vi "controllerMain.vi"(8 "error in (no error)":errorcluster, 10 "UserEvents in":refnum<class "UserEvents.lvclass">, 11 "Controller in":refnum<class "Controller.lvclass">) -> (0 "error out":errorcluster, 3 "Controller out":refnum<class "Controller.lvclass">)   [LabVIEW 2015, in "Controller.lvclass"]
uses:
  Controller.lvclass
  UserEvents/UserEvents.lvclass
  StateFactory/StateFactory.lvclass
  Typedefs/StateSelector.ctl
  Model/Model/Model.lvclass
  Context/Context.lvclass
  CommandFactory/CommandFactory.lvclass
  <userlib>/Common/SerialProtocols/SerialProtocolFactory/SerialProtocolFactory/SerialProtocolFactory.lvclass
  <userlib>/Common/SerialProtocols/SerialCommunicator/SerialCommunicator.lvclass
  Model/ILCTC/ILCTC.lvclass
  Model/PressureSensor/PressureSensor/PressureSensor.lvclass
  <userlib>/Common/SerialProtocols/SerialCommunicator/SerialCommunicator.lvclass/SerialCommunicator.ctl
  <userlib>/Common/ILC/ILC/ILC.lvclass/ILC.ctl
  Model/Model/Model.lvclass/Model.ctl
  UserEvents/UserEvents.lvclass/UserEvents.ctl
  Context/Context.lvclass/Context.ctl
  Command/Command.lvclass
  Typedefs/FAMTTypedefs.lvlib
  <userlib>/Common/ILC/ILC/ILC.lvclass
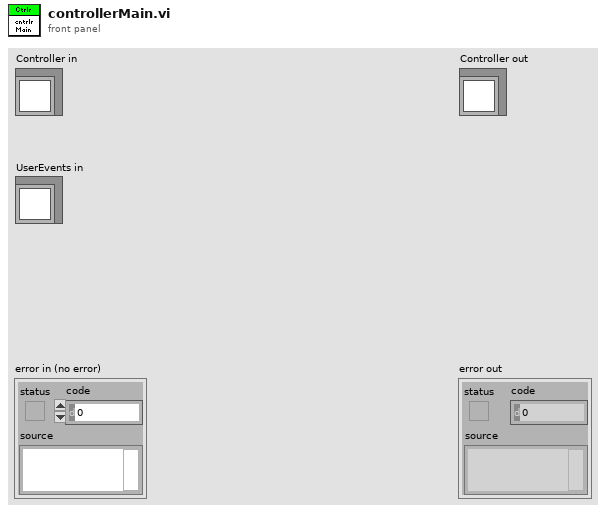
[diagram p1: front panel]
types:
  T1 = typedef "FAMTTypedefs.lvlib/StateSelector.ctl" = enum16{"OfflineState", "FaultState", "StandbyState", "DisabledState", "EnabledState", "WaitForUserInputState", "PerformOpenLoopScanState"}
  T2 = typedef "FAMTTypedefs.lvlib/SubDataEvents.ctl" = cluster{"Command":refnum<user-event>}
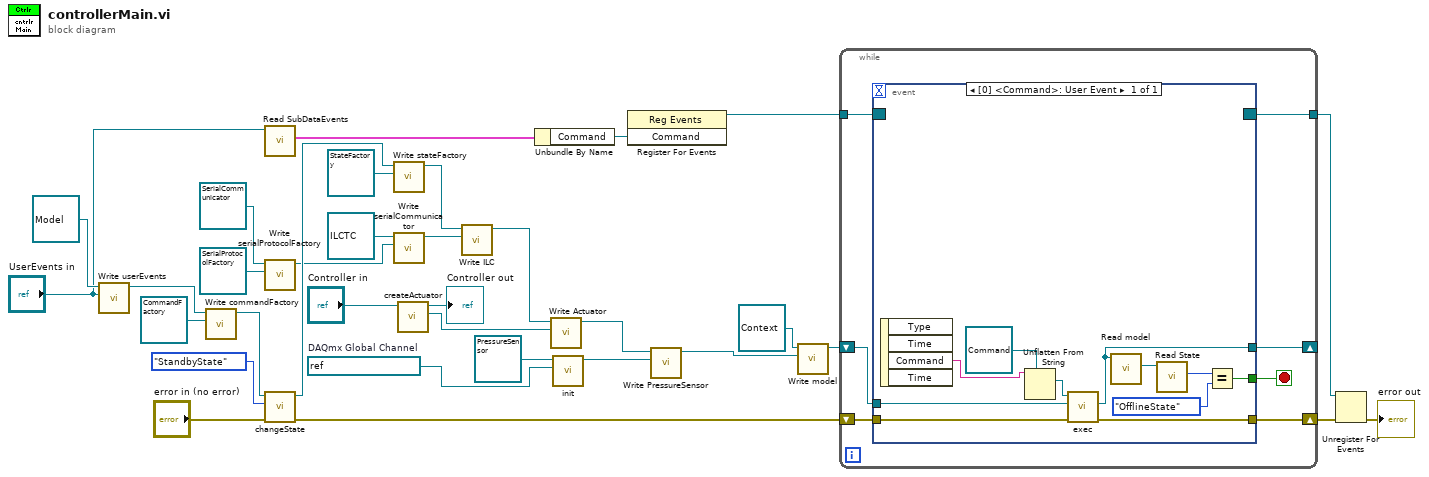
[diagram p0: block diagram]
diagram:
  w1 = refnum<k21> "PressureSensor1"  # DAQmx Global Channel
  n1 = call "Write userEvents.vi"("userEvents"="UserEvents in", "Model in"=refnum<class "Model.lvclass"> refnum) -> ("Model out"=w17:refnum<class "Model.lvclass">)  [unwired: 9 in]
  n2 = call "Write commandFactory.vi"("commandFactory"=refnum<class "CommandFactory.lvclass"> refnum ("CommandFactory.lvclass"), "Model in"=w17) -> ("Model out"=w15:refnum<class "Model.lvclass">)  [unwired: 9 in]
  n3 = call "Read SubDataEvents.vi"("UserEvents in"="UserEvents in") -> ("SubDataEvents"=w29:T2)  [unwired: 9 in, 1 out]
  n4 = call <userlib>:"Write serialProtocolFactory.vi"("serialProtocolFactory"=refnum<class "SerialProtocolFactory.lvclass"> refnum ("SerialCommFactory.lvclass"), "SerialCommunicator in"=refnum<class "SerialCommunicator.lvclass"> refnum ("SerialProtocols.lvlib:SerialCommunicator.lvclass")) -> ("SerialCommunicator out"=w11:refnum<class "SerialCommunicator.lvclass">)  [unwired: 9 in]
  n5 = call "changeState.vi"("error in (no error)"="error in (no error)", "State:"=StateSelector."StandbyState", "Model in"=w15) -> ("error out"=w25:errorcluster, "Model out"=w13:refnum<class "Model.lvclass">)  [unwired: 7 in]
  n6 = call "Write stateFactory.vi"("stateFactory"=refnum<class "StateFactory.lvclass"> refnum ("StateFactory.lvclass"), "Model in"=w13) -> ("Model out"=w20:refnum<class "Model.lvclass">)  [unwired: 9 in]
  n7 = call <userlib>:"Write serialCommunicator.vi"("serialCommunicator"=w11, "ILC in"=refnum<class "ILCTC.lvclass"> refnum ("ILC_TC.lvclass")) -> ("ILC out"=w6:refnum<class "ILCTC.lvclass">)  [unwired: 9 in]
  n8 = call "createActuator.vi"("Controller in"="Controller in") -> ("Actuator"=w8:refnum<class "IActuator.lvclass">, "Controller out"=→"Controller out":refnum<class "Controller.lvclass">)  [unwired: 8 in, 1 out]
  n9 = call "Write ILC.vi"("ilc"=w6, "Model in"=w20) -> ("Model out"=w7:refnum<class "Model.lvclass">)  [unwired: 9 in]
  n10 = Unbundle By Name(w29) -> ("Command"=w23:refnum<user-event>)
  n11 = call "Write Actuator.vi"("IActuator.lvclass"=w8, "Model in"=w7) -> ("Model out"=w4:refnum<class "Model.lvclass">)  [unwired: 9 in]
  n12 = call "init.vi"("Pressure Sensor 1"=w1, "PressureSensor in"=refnum<class "PressureSensor.lvclass"> refnum ("PressureSensor.lvclass")) -> ("PressureSensor out"=w2:refnum<class "PressureSensor.lvclass">)  [unwired: 8 in, 1 out]
  n13 = register-events(w23) -> (reference out=w28:refnum<event-registration>)  [unwired: 2 in, 1 out]
  n14 = call "Write PressureSensor.vi"("PressureSensor"=w2, "Model in"=w4) -> ("Model out"=w3:refnum<class "Model.lvclass">)  [unwired: 9 in]
  n15 = call "Write model.vi"("Model.lvclass"=w3, "Context in"=refnum<class "Context.lvclass"> refnum ("Context.lvclass")) -> ("Context out"=w31:refnum<class "Context.lvclass">)  [unwired: 9 in]
  n16 = while {
    shift-right: [w39] -> w26
    shift-left: w25 -> [w36]
    shift-right: [w38] -> _
    shift-left: w31 -> [w40]
    tunnel: w28 -> [w35]
    tunnel: [w34] -> w27
    stop <- w37 stop-if-true
    n17 = event shown="[0] <Command>: User Event" {
      selector: w35 -> [_]
      dyn-events: [_] -> w34
      timeout: _ -> [_]
      tunnel: w40 -> [w49]
      tunnel: [w46] -> w39
      tunnel: [w45] -> w38
      tunnel: [w44] -> w37
      tunnel: w36 -> [w42]
      event User Event {
        n18 = event-data() -> ("Command"=w41:string)  [unwired: 1 in, 3 out]
        n19 = Unflatten From String(type=refnum<class "Command.lvclass"> refnum ("Command.lvclass"), binary string=w41) -> (value=w50:refnum<class "Command.lvclass">)  [unwired: 3 in, 2 out]
        n20 = call-dynamic "exec.vi"("error in (no error)"=w42, "context"=w49, "Command in"=w50) -> ("error out"=w46:errorcluster, "context 2"=w45:refnum<class "Context.lvclass">)  [unwired: 6 in, 1 out]
        n21 = call "Read model.vi"("Context in"=w45) -> ("Model.lvclass"=w48:refnum<class "Model.lvclass">)  [unwired: 9 in, 1 out]
        n22 = call "Read State.vi"("Model in"=w48) -> ("state:"=w43:T1)  [unwired: 9 in, 1 out]
        n23 = Equal?(x=w43, y=StateSelector."OfflineState") -> (x = y?=w44:bool)
      }
    }
  }
  n24 = Unregister For Events(event registration refnum=w27, error in=w26) -> (error out=→"error out":errorcluster)
